vi "ECEF_2_LLA(SubVI).vi"(11 "p_new":dbl[](array[numeric])) -> (1 "lon":dbl, 2 "latd":dbl, 3 "altd":dbl)   [LabVIEW 2017]
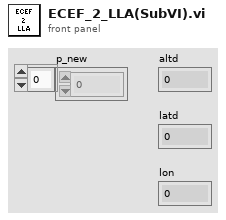
[diagram p1: front panel]
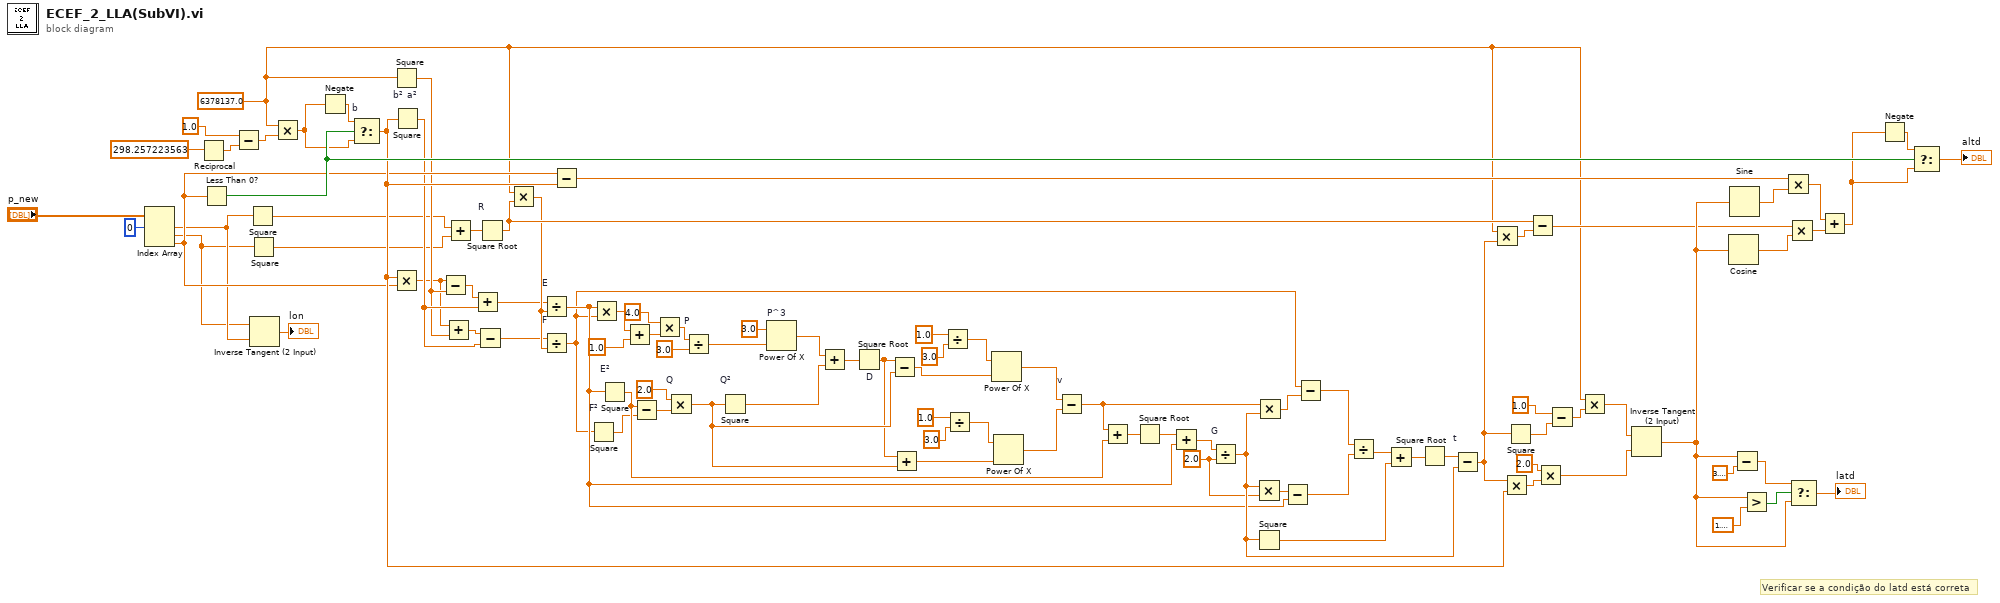
[diagram p0: block diagram]
diagram:
  w53 = 2.0 ("y")
  w74 = 6378137.0
  # "Verificar se a condição do latd está correta"
  n1 = Index Array(array="p_new", index #1=0 ("index")) -> (element #1=w71:dbl, element #2=w70:dbl, element #3=w77:dbl)  [unwired: 2 in]
  n2 = Reciprocal(x=298.257223563) -> (1/x=w2:dbl)
  n3 = Less Than 0?(x=w77) -> (x < 0?=w88:bool)
  n4 = Subtract(x=1.0, y=w2) -> (x-y=w4:dbl)
  n5 = Square(x=w71) -> (x^2=w10:dbl)
  n6 = Square(x=w70) -> (x^2=w9:dbl)
  n7 = Inverse Tangent (2 Input)(1:w71, 2:w70) -> (0:→"lon":dbl)
  n8 = Multiply(x=w74, y=w4) -> (x*y=w6:dbl)
  n9 = Negate(x=w6) -> (-x=w5:dbl)
  n10 = Select "b"(t=w5, s=w88, f=w6) -> (s? t:f=w78:dbl)
  n11 = Square "a²"(x=w74) -> (x^2=w15:dbl)
  n12 = Multiply(x=w78, y=w77) -> (x*y=w14:dbl)
  n13 = Square "b²"(x=w78) -> (x^2=w17:dbl)
  n14 = Subtract(x=w14, y=w15) -> (x-y=w12:dbl)
  n15 = Add(x=w14, y=w15) -> (x+y=w16:dbl)
  n16 = Add(x=w10, y=w9) -> (x+y=w11:dbl)
  n17 = Add(x=w12, y=w17) -> (x+y=w13:dbl)
  n18 = Subtract(x=w16, y=w17) -> (x-y=w18:dbl)
  n19 = Square Root "R"(x=w11) -> (sqrt(x)=w76:dbl)
  n20 = Multiply(x=w74, y=w76) -> (x*y=w19:dbl)
  n21 = Divide "E"(x=w13, y=w19) -> (x/y=w55:dbl)
  n22 = Divide "F"(x=w18, y=w19) -> (x/y=w52:dbl)
  n23 = Subtract(x=w77, y=w78) -> (x-y=w83:dbl)
  n24 = Square "F²"(x=w52) -> (x^2=w26:dbl)
  n25 = Multiply(x=w55, y=w52) -> (x*y=w20:dbl)
  n26 = Square "E²"(x=w55) -> (x^2=w46:dbl)
  n27 = Add(x=w20, y=1.0) -> (x+y=w22:dbl)
  n28 = Subtract(x=w46, y=w26) -> (x-y=w27:dbl)
  n29 = Multiply(x=4.0, y=w22) -> (x*y=w24:dbl)
  n30 = Multiply "Q"(x=2.0, y=w27) -> (x*y=w42:dbl)
  n31 = Divide "P"(x=w24, y=3.0) -> (x/y=w29:dbl)
  n32 = Square "Q²"(x=w42) -> (x^2=w32:dbl)
  n33 = Power Of X "P^3"(1:w29, 2:3.0 ("y")) -> (0:w31:dbl)
  n34 = Add(x=w31, y=w32) -> (x+y=w33:dbl)
  n35 = Square Root "D"(x=w33) -> (sqrt(x)=w41:dbl)
  n36 = Subtract(x=w41, y=w42) -> (x-y=w34:dbl)
  n37 = Add(x=w41, y=w42) -> (x+y=w43:dbl)
  n38 = Divide(x=1.0, y=3.0) -> (x/y=w37:dbl)
  n39 = Divide(x=1.0, y=3.0) -> (x/y=w38:dbl)
  n40 = Power Of X(1:w34, 2:w37) -> (0:w44:dbl)
  n41 = Power Of X(1:w43, 2:w38) -> (0:w45:dbl)
  n42 = Subtract "v"(x=w44, y=w45) -> (x-y=w50:dbl)
  n43 = Add(x=w50, y=w46) -> (x+y=w47:dbl)
  n44 = Square Root(x=w47) -> (sqrt(x)=w48:dbl)
  n45 = Add(x=w48, y=w55) -> (x+y=w49:dbl)
  n46 = Divide "G"(x=w49, y=w53) -> (x/y=w62:dbl)
  n47 = Multiply(x=w62, y=w53) -> (x*y=w54:dbl)
  n48 = Square(x=w62) -> (x^2=w59:dbl)
  n49 = Multiply(x=w50, y=w62) -> (x*y=w51:dbl)
  n50 = Subtract(x=w54, y=w55) -> (x-y=w57:dbl)
  n51 = Subtract(x=w52, y=w51) -> (x-y=w56:dbl)
  n52 = Divide(x=w56, y=w57) -> (x/y=w58:dbl)
  n53 = Add(x=w58, y=w59) -> (x+y=w60:dbl)
  n54 = Square Root(x=w60) -> (sqrt(x)=w61:dbl)
  n55 = Subtract "t"(x=w61, y=w62) -> (x-y=w73:dbl)
  n56 = Multiply(x=w74, y=w73) -> (x*y=w75:dbl)
  n57 = Multiply(x=w73, y=w78) -> (x*y=w66:dbl)
  n58 = Square(x=w73) -> (x^2=w64:dbl)
  n59 = Subtract(x=w76, y=w75) -> (x-y=w79:dbl)
  n60 = Multiply(x=2.0 ("y"), y=w66) -> (x*y=w68:dbl)
  n61 = Subtract(x=1.0 ("y"), y=w64) -> (x-y=w65:dbl)
  n62 = Multiply(x=w74, y=w65) -> (x*y=w69:dbl)
  n63 = Inverse Tangent (2 Input)(1:w68, 2:w69) -> (0:w93:dbl)
  n64 = Cosine(x=w93) -> (cos(x)=w80:dbl)
  n65 = Sine(x=w93) -> (sin(x)=w82:dbl)
  n66 = Subtract(x=w93, y=3.141592653589793) -> (x-y=w92:dbl)
  n67 = Greater?(x=w93, y=1.5707963267948966) -> (0:w89:bool)
  n68 = Multiply(x=w83, y=w82) -> (x*y=w84:dbl)
  n69 = Multiply(x=w79, y=w80) -> (x*y=w81:dbl)
  n70 = Select(t=w92, s=w89, f=w93) -> (s? t:f=→"latd":dbl)
  n71 = Add(x=w84, y=w81) -> (x+y=w86:dbl)
  n72 = Negate(x=w86) -> (-x=w85:dbl)
  n73 = Select(t=w85, s=w88, f=w86) -> (s? t:f=→"altd":dbl)
